vi "main().vi"() -> ()   [LabVIEW 2016]
uses:
  <vilib>/LabVIEW Interface for Arduino/LabVIEW Interface for Arduino.lvlib
panel:
  in  "numero du port (capteur lumière)":u8
  out "indicateur de lumière :":bool
  out "intensité de la lumière en temps réel :":dbl(knob) scale=0.0..100.0
  in  "seuil de lumière :":dbl
  in  "numero du port (capteur température)":u8
  in  "baude rate de la carte":u32
  in  "numero port de communication (pc-->carte)":refnum<visa-resource-name>
  in  "seuil de la temperature :":dbl
  out "indicateur de température :":bool
  out "température en temps réel:":dbl(slide) scale=0.0..100.0
  # "--> ici vous trouverez les indicateurs de lumière :"
  # "--> ici vous trouvez les indicateurs de température :"
  # "veuillez choisisser un seuil entre 0 et 100 :"
  # "veuillez choisissez un seuil entre 0 et 100 :"
  # "--> veuillez configurer votre carte ci dessous :"
  # "utilisez une resistance 10K"
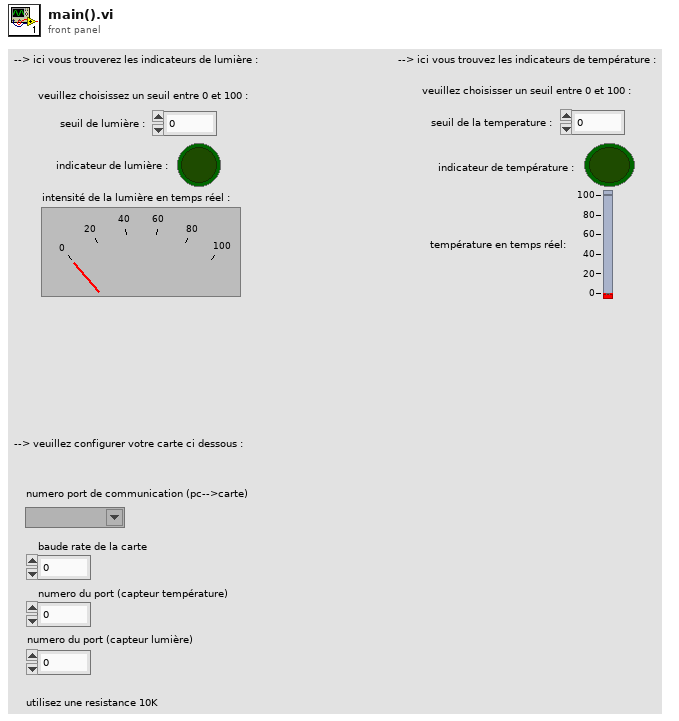
[diagram p1: front panel]
types:
  T1 = typedef "LabVIEW Interface for Arduino.lvlib/Arduino Resource.ctl" = cluster{"VISA resource":refnum<visa-resource-name>, "Board Type":T2, "Connection Type":enum8{"USB / Serial"}, "Bytes Per Packet (15)":u8}
  T2 = typedef "LabVIEW Interface for Arduino.lvlib/Board Type.ctl" = enum16{"Uno", "Dimuelanove w/Atmega 328", "Mega 2560"}
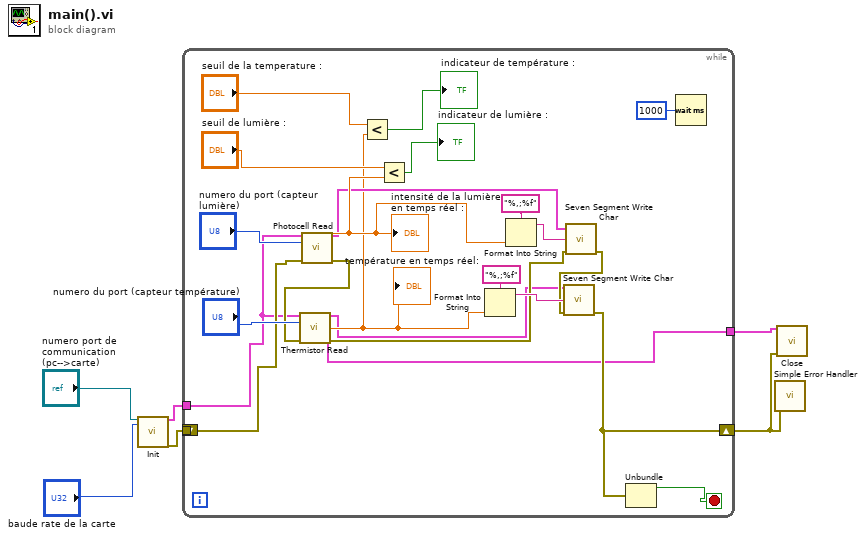
[diagram p0: block diagram]
diagram:
  n1 = call <vilib>:"Init.vi"("VISA resource"="numero port de communication (pc-->carte)", "Baud Rate (115200)"="baude rate de la carte") -> ("Arduino Resource"=w5:T1, "error out"=w1:errorcluster)  [unwired: 16 in]
  n2 = while {
    tunnel: w1 -> [w23]
    tunnel: w5 -> [w12]
    tunnel: [w7] -> w2
    shift-right: [w11] -> w3
    shift-left: w1 -> [_]
    stop <- w18 stop-if-true
    n3 = call <vilib>:"Photocell Read.vi"("Arduino Resource"=w12, "Photo Cell Pin (0)"="numero du port (capteur lumière)", "error in"=w23) -> ("Arduino Resource"=w10:T1, "Light Intensity (0 - 100)"=w16:dbl, "error out"=w22:errorcluster)  [unwired: 10 in]
    "intensité de la lumière en temps réel :" <- w16
    n4 = call <vilib>:"Thermistor Read.vi"("Arduino Resource"=w12, "Thermistor AI Pin (0)"="numero du port (capteur température)", "error in"=w22) -> ("Arduino Resource"=w7:T1, "Temperature"=w8:dbl, "error out"=w15:errorcluster)  [unwired: 10 in]
    "température en temps réel:" <- w8
    n5 = Less?(x="seuil de la temperature :", y=w8) -> (x < y?=→"indicateur de température :":bool)
    n6 = Less?(x="seuil de lumière :", y=w16) -> (x < y?=→"indicateur de lumière :":bool)
    n7 = Format Into String(format string="%,;%f", w8) -> (resulting string=w25:string)  [unwired: 2 in, 1 out]
    n8 = Format Into String(format string="%,;%f", w16) -> (resulting string=w13:string)  [unwired: 2 in, 1 out]
    n9 = call <vilib>:"Seven Segment Write Char.vi"("Arduino Resource"=w10, "Character"=w13, "error in (no error)"=w15) -> ("error out"=w14:errorcluster)  [unwired: 11 in, 1 out]
    n10 = call <vilib>:"Seven Segment Write Char.vi"("Arduino Resource"=w7, "Character"=w25, "error in (no error)"=w14) -> ("error out"=w11:errorcluster)  [unwired: 11 in, 1 out]
    n11 = Unbundle(w11) -> ("status"=w18:bool)  [unwired: 2 out]
    n12 = Wait (ms)(milliseconds to wait=u32 1000) -> ()  [unwired: 1 out]
  }
  n13 = call <vilib>:"Simple Error Handler.vi"("error in (no error)"=w3) -> ()  [unwired: 4 in, 5 out]
  n14 = call <vilib>:"Close.vi"("Arduino Resource"=w2, "error in"=w3) -> ()  [unwired: 13 in, 1 out]
